vi "mysql_database_insert.vi"(1 "SQL query":string) -> (0 "error out":errorcluster)   [LabVIEW 2023]
uses:
  <vilib>/addons/database/Connection.llb/DB Tools Open Connec (Path).vi
  <vilib>/addons/database/Connection.llb/Conn Execute.vi
  <vilib>/addons/database/Recordset.llb/Rec Fetch Recordset Data (R).vi
  <vilib>/addons/database/Recordset.llb/Rec Destroy - Connection.vi
  <vilib>/addons/database/NI_Database_API.lvlib
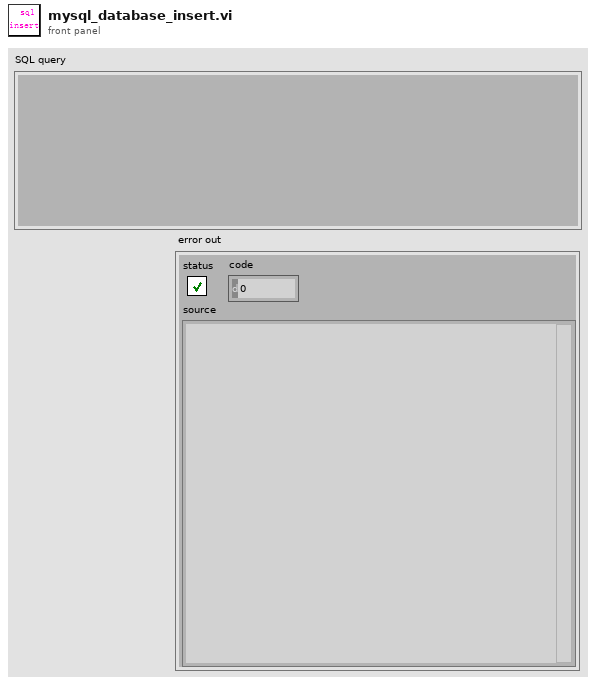
[diagram p1: front panel]
types:
  T1 = typedef "NI_Database_API.lvlib/Conn ObjectReference.ctl" = refnum<k1>
  T2 = typedef "NI_Database_API.lvlib/Rec ObjectReference.ctl" = refnum<k1>
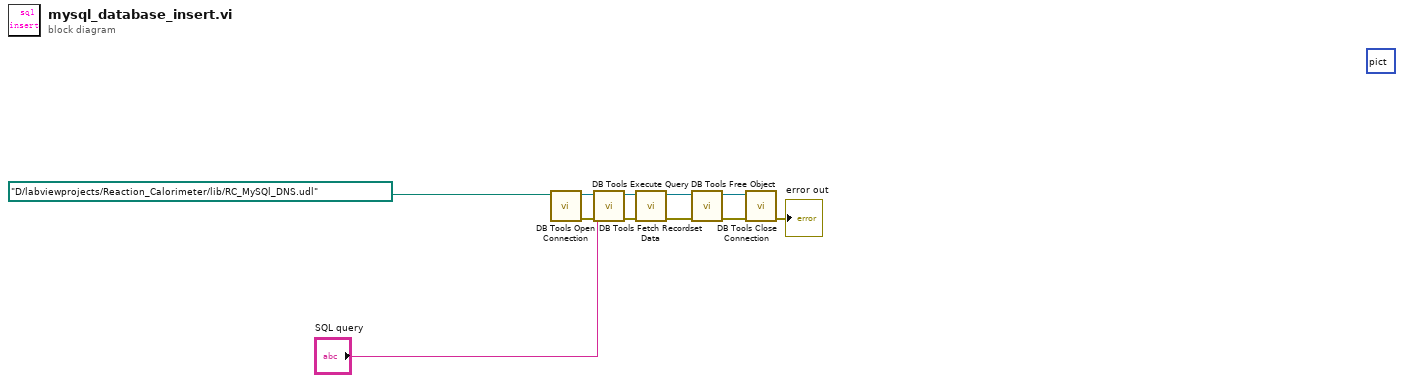
[diagram p0: block diagram]
diagram:
  (unwired) picture bytes[5395230] ("二维图片")
  n1 = call-poly <vilib>:"DB Tools Open Connection.vi"("connection information"=path "D:/labviewprojects/Reaction_Calorimeter/lib/RC_MySQl_DNS.udl") -> ("error out"=w9:errorcluster, "connection reference"=w10:T1)  [unwired: 7 in]
  n2 = call-poly <vilib>:"DB Tools Execute Query.vi"("error in (no error)"=w9, "SQL query"="SQL query", "connection reference"=w10) -> ("error out"=w3:errorcluster, "recordset reference"=w6:T2)  [unwired: 5 in]
  n3 = call-poly <vilib>:"DB Tools Fetch Recordset Data.vi"("error in (no error)"=w3, "recordset reference"=w6) -> ("error out"=w4:errorcluster, "recordset reference out"=w5:T2)  [unwired: 3 in, 1 out]
  n4 = call-poly <vilib>:"DB Tools Free Object.vi"("error in (no error)"=w4, "recordset reference"=w5) -> ("error out"=w7:errorcluster, "connection reference"=w8:T1)  [unwired: 8 in]
  n5 = call <vilib>:"DB Tools Close Connection.vi"("error in (no error)"=w7, "connection reference"=w8) -> ("error out"=→"error out":errorcluster)  [unwired: 5 in]
